vi "zmq_recv_timeout.vi"(4 "error in":errorcluster, 5 "timeout (ms)":u32=500, 7 "socket in":refnum<class "zmq_socket.lvclass">) -> (0 "error out":errorcluster, 1 "timeout?":bool, 2 "parts":string[](array[string]), 3 "socket out":refnum<class "zmq_socket.lvclass">)   [LabVIEW 2019, in "zeromq.lvlib" / "zmq_socket.lvclass"]
doc: "An implementation of \"receive with timeout\" functionality, returning an array of strings as per zmq_recv_multi. This VI is provided as a development \"crutch\" and is against the ZeroMQ philosophy but is highly convenient in some situations.\n\nPolls <b>socket in</b> periodically every <b>poll interval</b> milliseconds until a message has been received, or <b>timeout</b> milliseconds elapses since the start of the call. Aborts on error.\n\nDetailed API documentation: http://api.zeromq.org/3-2:zmq-poll"
uses:
  zmq_socket.lvclass
  zmq_socket.lvclass/zmq_socket.ctl
  <vilib>/Utility/error.llb/Error Cluster From Error Code.vi
  zeromq.lvlib
panel:
  # "ØMQ"
  # "labview"
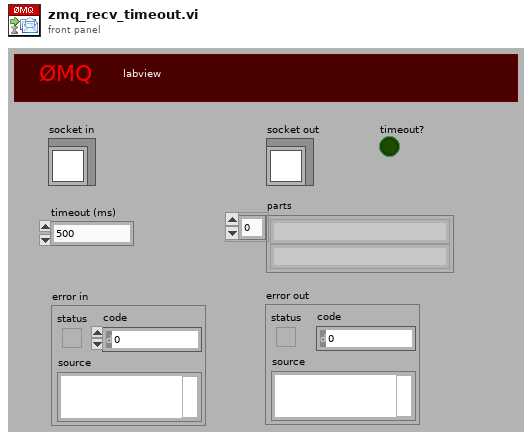
[diagram p1: front panel]
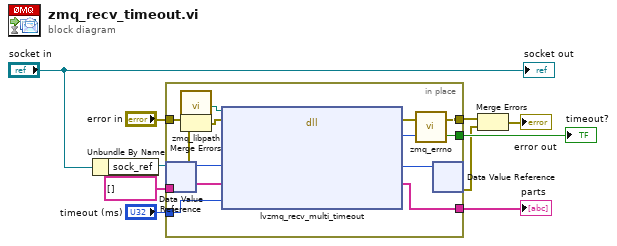
[diagram p0: block diagram]
diagram:
  n1 = Unbundle By Name("socket in") -> ("sock_ref"=w3:refnum<data-value>)
  n2 = in-place {
    in-place-border: string[] [] ("parts") -> [w23]
    in-place-border: [w22] -> w9
    in-place-border: "timeout (ms)" -> [w21]
    in-place-border: "error in" -> [w20]
    in-place-border: [w17] -> w6
    in-place-border: [w16] -> w5
    n3 = in-place-dvr #1(w3) -> (w15:u64, w11:errorcluster)
    n4 = call "zmq_libpath.vi"() -> ("path"=w13:path)
    n5 = Merge Errors(w20, w11) -> (w12:errorcluster)
    n6 = dll-call lib="?" fn="lvzmq_recv_multi_timeout" ("zmq_labview.dll:lvzmq_socket")(path in=w13, error in=w12, "sock_obj"=w15, "data"=w23, "timeout"=w21) -> (error out=w19:errorcluster, "return type"=w18:i32, "sock_obj"=w14:u64, "data"=w22:string[])  [unwired: 4 in, 1 out]
    n7 = call "zmq_errno.vi"("retval"=w18, "error in"=w19) -> ("again?"=w16:bool, "error out"=w17:errorcluster)
    n8 = in-place-dvr #1(w14) -> (w1:errorcluster)  [unwired: 1 out]
  }
  "parts" <- w9
  "timeout?" <- w5
  n9 = Merge Errors(w6, w1) -> (→"error out":errorcluster)
  "socket out" <- "socket in"
